vi "init runtime test.vi"() -> (0 "no error":errorcluster, 2 "tags found":bool, 3 "expected execution settings":bool)   [LabVIEW 2020, in "dds tests.lvlib"]
uses:
  dds tests.lvlib
  module/execution/dds runtime.lvclass
  <vilib>/NI/Tag Bus/tag/tag descriptor.lvclass/tag descriptor.ctl
  <vilib>/NI/Tag Bus Module Framework/channel/TBM channel.lvclass/TBM channel.ctl
  <vilib>/NI/Tag Bus/tag/read tag name.vi
  <vilib>/NI/Tag Bus/tag/read data type.vi
  <vilib>/NI/Tag Bus Module Framework/channel/Read channel classification.vi
  module/configuration/dds configuration.lvclass
  C:/Program Files (x86)/National Instruments/LabVIEW 2020/vi.lib/NI/Tag Bus Module Framework/module configuration/TBM module configuration.lvclass
  <vilib>/NI/Tag Bus Module Framework/channel/TBM channel.lvclass
  C:/Program Files (x86)/National Instruments/LabVIEW 2020/vi.lib/NI/Tag Bus/tag/tag descriptor.lvclass
  <vilib>/NI/Tag Bus/dictionary/data dictionary.lvclass
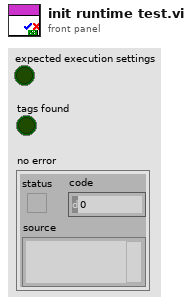
[diagram p1: front panel]
types:
  T1 = typedef "TBM channel.lvclass/data tables.ctl" = cluster{"input data":T2, "processing parameter":T2, "processing result":T2, "output data":T2}
  T2 = typedef "tag bus.lvlib/dictionary table pair.ctl" = cluster{"data dictionary":refnum<class "data dictionary.lvclass">, "data table":T3}
  T3 = typedef "tag bus.lvlib/data table.lvlib/data table.ctl" = cluster{"Double":dbl[], "Single":sgl[], "I64":i64[], "I32":i32[], "I16":i16[], "I8":i8[], "U64":u64[], "U32":u32[], "U16":u16[], "U8":u8[], "Boolean":bool[], "String":string[], "Array of Double":cluster{"DBL Array":dbl[]}[], "Array of Single":cluster{"SGL Array":sgl[]}[], "Array of I64":cluster{"I64 Array":i64[]}[], "Array of I32":cluster{"I32 Array":i32[]}[], "Array of I16":cluster{"I16 Array":i16[]}[], "Array of I8":cluster{"I8 Array":i8[]}[], "Array of U64":cluster{"U64 Array":u64[]}[], "Array of U32":cluster{"U32 Array":u32[]}[], "Array of U16":cluster{"U16 Array":u16[]}[], "Array of U8":cluster{"U8 Array":u8[]}[], "Array of Boolean":cluster{"Boolean Array":bool[]}[], "Array of String":cluster{"String Array":string[]}[]}
  T4 = typedef "TBM module execution interface.lvclass/execution settings.ctl" = cluster{"reads inputs":bool, "processes data":bool, "writes outputs":bool}
  T5 = typedef "tag bus.lvlib/tag descriptor.lvclass/Data Type.ctl" = enum16{"Double", "Single", "I64", "I32", "I16", "I8", "U64", "U32", "U16", "U8", "Boolean", "String", "Array of Double", "Array of Single", "Array of I64", "Array of I32", "Array of I16", "Array of I8", "Array of U64", "Array of U32", "Array of U16", "Array of U8", "Array of Boolean", "Array of String"}
  T6 = typedef "TBM channel.lvclass/channel classification.ctl" = enum16{"input data", "output data", "processing parameter", "processing result"}
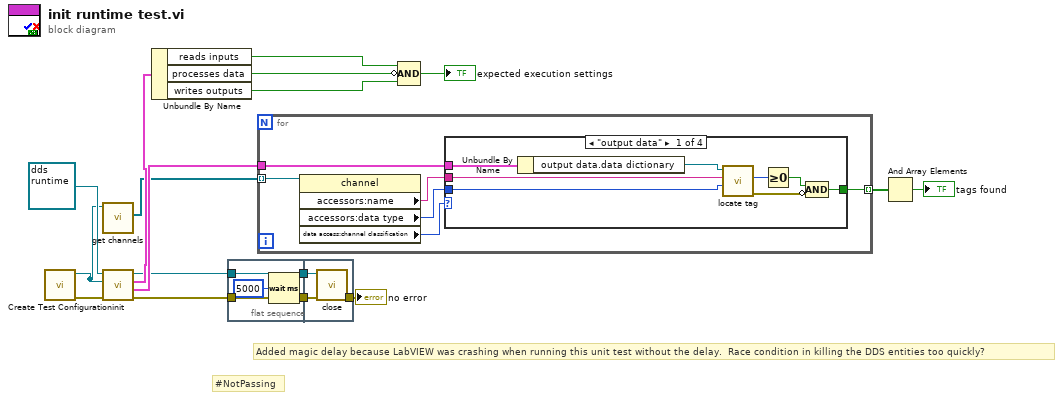
[diagram p0: block diagram]
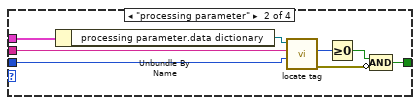
[diagram p2: hidden frame]
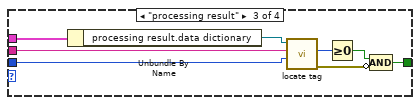
[diagram p3: hidden frame]
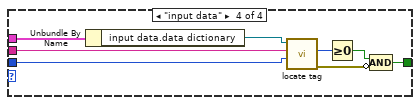
[diagram p4: hidden frame]
diagram:
  # "Added magic delay because LabVIEW was crashing when running this unit test without the delay.  Race condition in killing the DDS entities too quickly?"
  # "#NotPassing"
  n1 = call "Create Test Configuration.vi"() -> ("error out"=w5:errorcluster, "module"=w4:refnum<class "dds configuration.lvclass">)  [unwired: 6 in, 4 out]
  n2 = call-dynamic "get channels.vi"("dds configuration in"=w4) -> ("channels"=w3:refnum<class "TBM channel.lvclass">[])  [unwired: 9 in, 1 out]
  n3 = call-dynamic "init.vi"("error in"=w5, "TBM module configuration in"=w4, "dds runtime in"=refnum<class "dds runtime.lvclass"> refnum ("tag bus configurable plugin module")) -> ("error out"=w9:errorcluster, "data allocations"=w17:T1, "execution settings"=w16:T4, "dds runtime out"=w8:refnum<class "dds runtime.lvclass">)  [unwired: 5 in]
  n4 = Unbundle By Name(w16) -> ("reads inputs"=w15:bool, "processes data"=w13:bool, "writes outputs"=w14:bool)
  n5 = flat-sequence {
    tunnel: w8 -> [w19]
    tunnel: w9 -> [w20]
    tunnel: [w20] -> w2
    tunnel: [w19] -> w1
    tunnel: [w21] -> w7
    tunnel: w2 -> [w23]
    tunnel: w1 -> [w22]
    frame #0 {
      n6 = Wait (ms)(milliseconds to wait=u32 5000) -> ()  [unwired: 1 out]
    }
    frame #1 {
      n7 = call-dynamic "close.vi"("error in"=w23, "dds runtime in"=w22) -> ("error out"=w21:errorcluster)  [unwired: 9 in]
    }
  }
  n8 = for {
    tunnel: w17 -> [w29]
    tunnel: w3 -> [w28] mode=indexing
    tunnel: [w27] -> w11 mode=indexing
    n9 = property class="channel"(reference=w28) -> ("accessors:name"=w24:string, "accessors:data type"=w25:T5, "data access:channel classification"=w26:T6)  [unwired: 1 in, 2 out]
    n10 = case shown="\"output data\"" w26 {
      tunnel: w29 -> [w37 w45 w53 w61]
      tunnel: w25 -> [w35 w43 w51 w59]
      tunnel: w24 -> [w34 w42 w50 w58]
      tunnel: [w30 w38 w46 w54] -> w27
      frame "output data" {
        n11 = Unbundle By Name(w37) -> ("output data.data dictionary"=w36:refnum<class "data dictionary.lvclass">)
        n12 = call <vilib>:"locate tag.vi"("data type"=w35, "name"=w34, "data dictionary in"=w36) -> ("error out"=w31:errorcluster, "index"=w33:i32)  [unwired: 6 in, 1 out]
        n13 = Greater Or Equal To 0?(x=w33) -> (x >= 0?=w32:bool)
        n14 = Compound Arithmetic op=AND(w32, invert w31) -> (w30:bool)
      }
      frame "processing parameter" {
        n15 = Unbundle By Name(w45) -> ("processing parameter.data dictionary"=w44:refnum<class "data dictionary.lvclass">)
        n16 = call <vilib>:"locate tag.vi"("data type"=w43, "name"=w42, "data dictionary in"=w44) -> ("error out"=w39:errorcluster, "index"=w41:i32)  [unwired: 6 in, 1 out]
        n17 = Greater Or Equal To 0?(x=w41) -> (x >= 0?=w40:bool)
        n18 = Compound Arithmetic op=AND(w40, invert w39) -> (w38:bool)
      }
      frame "processing result" {
        n19 = Unbundle By Name(w53) -> ("processing result.data dictionary"=w52:refnum<class "data dictionary.lvclass">)
        n20 = call <vilib>:"locate tag.vi"("data type"=w51, "name"=w50, "data dictionary in"=w52) -> ("error out"=w47:errorcluster, "index"=w49:i32)  [unwired: 6 in, 1 out]
        n21 = Greater Or Equal To 0?(x=w49) -> (x >= 0?=w48:bool)
        n22 = Compound Arithmetic op=AND(w48, invert w47) -> (w46:bool)
      }
      frame "input data" {
        n23 = Unbundle By Name(w61) -> ("input data.data dictionary"=w60:refnum<class "data dictionary.lvclass">)
        n24 = call <vilib>:"locate tag.vi"("data type"=w59, "name"=w58, "data dictionary in"=w60) -> ("error out"=w55:errorcluster, "index"=w57:i32)  [unwired: 6 in, 1 out]
        n25 = Greater Or Equal To 0?(x=w57) -> (x >= 0?=w56:bool)
        n26 = Compound Arithmetic op=AND(w56, invert w55) -> (w54:bool)
      }
    }
  }
  n27 = Compound Arithmetic op=AND(w15, invert w13, w14) -> (→"expected execution settings":bool)
  n28 = And Array Elements(Boolean array=w11) -> (logical AND=→"tags found":bool)
  "no error" <- w7
